vi "TCP Write with Length (TCP Cluster).vi"(8 "error in (no error)":errorcluster, 9 "timeout ms (25000)":i32, 10 "?":T1={"Datatype"=enum."Message", "String"="Hey, geh weg!"}, 11 "connection ID":refnum<k5>) -> (0 "error out":errorcluster, 3 "connection ID out":refnum<k5>)   [LabVIEW 2017]
uses:
  TypeDefinitions/TCP Cluster.ctl
  TypeDefinitions/TCP Commands.ctl
panel:
  out "length":i32
  # "Flatten String und ergänzen um \nString Länge statt einfachem \"Write\""
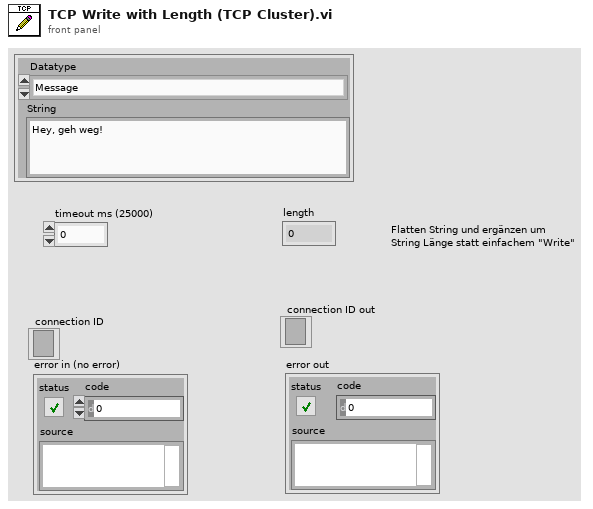
[diagram p1: front panel]
types:
  T1 = typedef "TCP Cluster.ctl" = cluster{"Datatype":T2, "String":string}
  T2 = typedef "TCP Commands.ctl" = enum16{"Timeout", "Log", "Message", "ManualDrive", "Stop", "Command"}
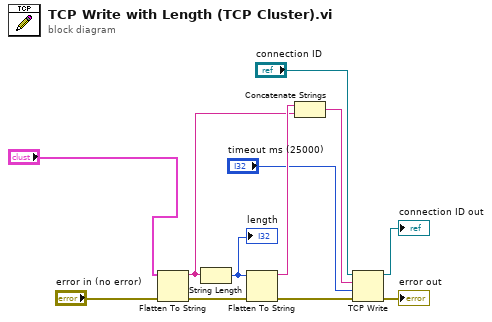
[diagram p0: block diagram]
diagram:
  n1 = Flatten To String(anything="?", error in (no error)="error in (no error)") -> (data string=w10:string, error out=w9:errorcluster)  [unwired: 2 in, 1 out]
  n2 = String Length(string=w10) -> (length=w12:i32)
  "length" <- w12
  n3 = Flatten To String(anything=w12, error in (no error)=w9) -> (data string=w11:string, error out=w6:errorcluster)  [unwired: 2 in, 1 out]
  n4 = Concatenate Strings(w11, w10) -> (w8:string)
  n5 = TCP Write(connection ID="connection ID", data in=w8, error in (no error)=w6, 9:"timeout ms (25000)") -> (connection ID out=→"connection ID out":refnum<k5>, error out=→"error out":errorcluster)  [unwired: 1 out]
